vi "SOC_FM Settings Dialog.vi"(8 "error in (no error)":errorcluster, 11 "User Specified":T1={"Hardware Configuration"={"HW Refnum <Replace Me>"="", "Signal Type <Replace Me>"=enum."Sine Wave"}, "Analysis Configuration"={"Statistics"=TRUE}, "New Data Behavior"=enum."Replace", "Calc PPL Path"=path "", "Calc Plugin Class Qualified Name"="", "Calc Configuration String"=""}) -> (0 "error out":errorcluster, 2 "UI Refresh Needed?":bool, 3 "User Specified 2":T1={"Hardware Configuration"={"HW Refnum <Replace Me>"="", "Signal Type <Replace Me>"=enum."Sine Wave"}, "Analysis Configuration"={"Statistics"=TRUE}, "New Data Behavior"=enum."Replace", "Calc PPL Path"=path "", "Calc Plugin Class Qualified Name"="", "Calc Configuration String"=""})   [LabVIEW 2015]
doc: "Dialog for selecting user specified settings."
uses:
  controls/SOC_FM User Specified Data.ctl
  controls/SOC_FM HW Configuration.ctl
  controls/SOC_FM Simulated Signal Type.ctl
  controls/SOC_FM Analysis Configuration.ctl
  controls/SOC_FM New Data Behavior.ctl
panel:
  in  "Calc Configuration String":string
  in  "Calc Plugin Class Qualified Name":string
  in  "Calc PPL Path":path
  in  "Signal Type":u16(ring) items=["Sine Wave", "Square Wave"]
  in  "New Data Behavior":u16(ring) items=["Replace", "Overlay", "Append"]
  in  "Cancel Button":bool
  in  "OK Button":bool
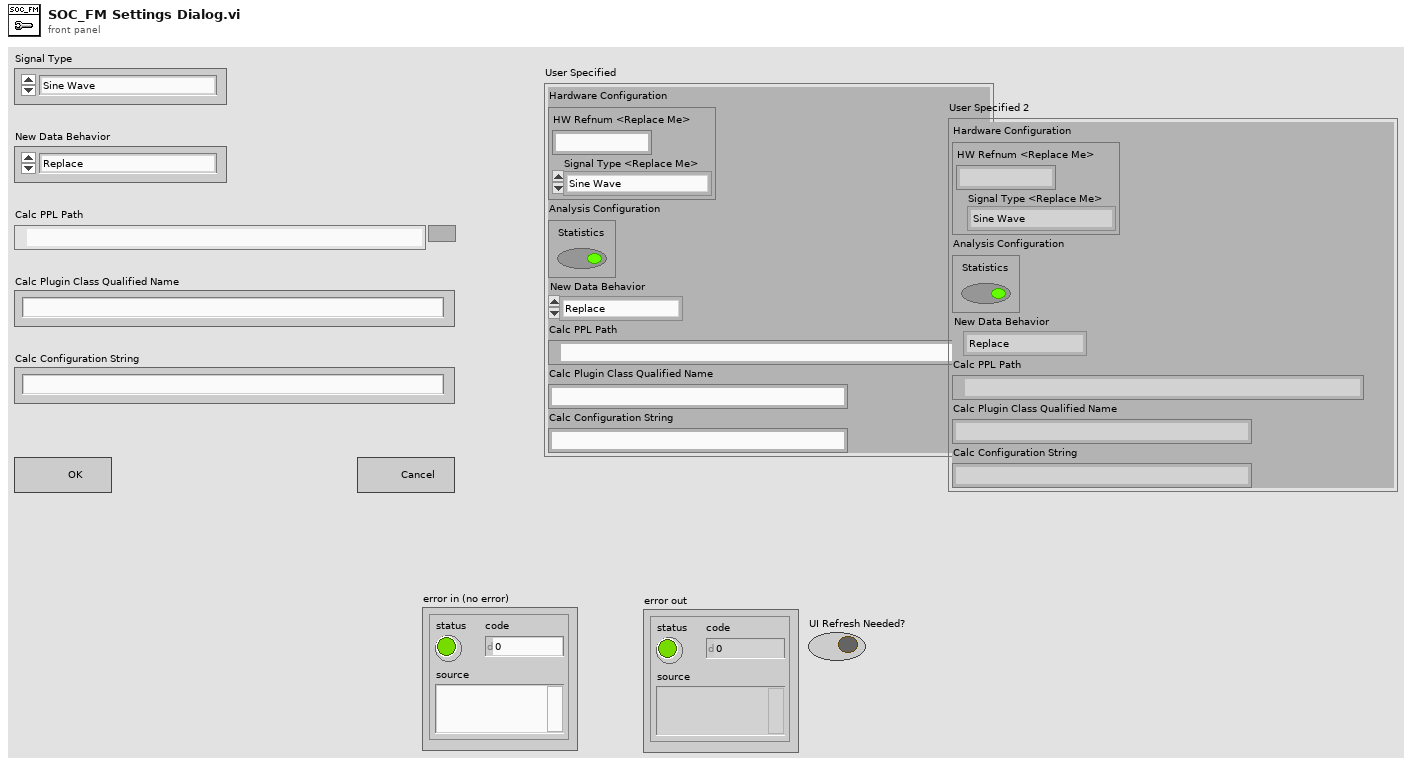
[diagram p1: front panel]
types:
  T1 = typedef "SOC_FM User Specified Data.ctl" = cluster{"Hardware Configuration":T2, "Analysis Configuration":T4, "New Data Behavior":T5, "Calc PPL Path":path, "Calc Plugin Class Qualified Name":string, "Calc Configuration String":string}
  T2 = typedef "SOC_FM HW Configuration.ctl" = cluster{"HW Refnum <Replace Me>":string, "Signal Type <Replace Me>":T3}
  T3 = typedef "SOC_FM Simulated Signal Type.ctl" = enum16{"Sine Wave", "Square Wave"}
  T4 = typedef "SOC_FM Analysis Configuration.ctl" = cluster{"Statistics":bool}
  T5 = typedef "SOC_FM New Data Behavior.ctl" = enum16{"Replace", "Overlay", "Append"}
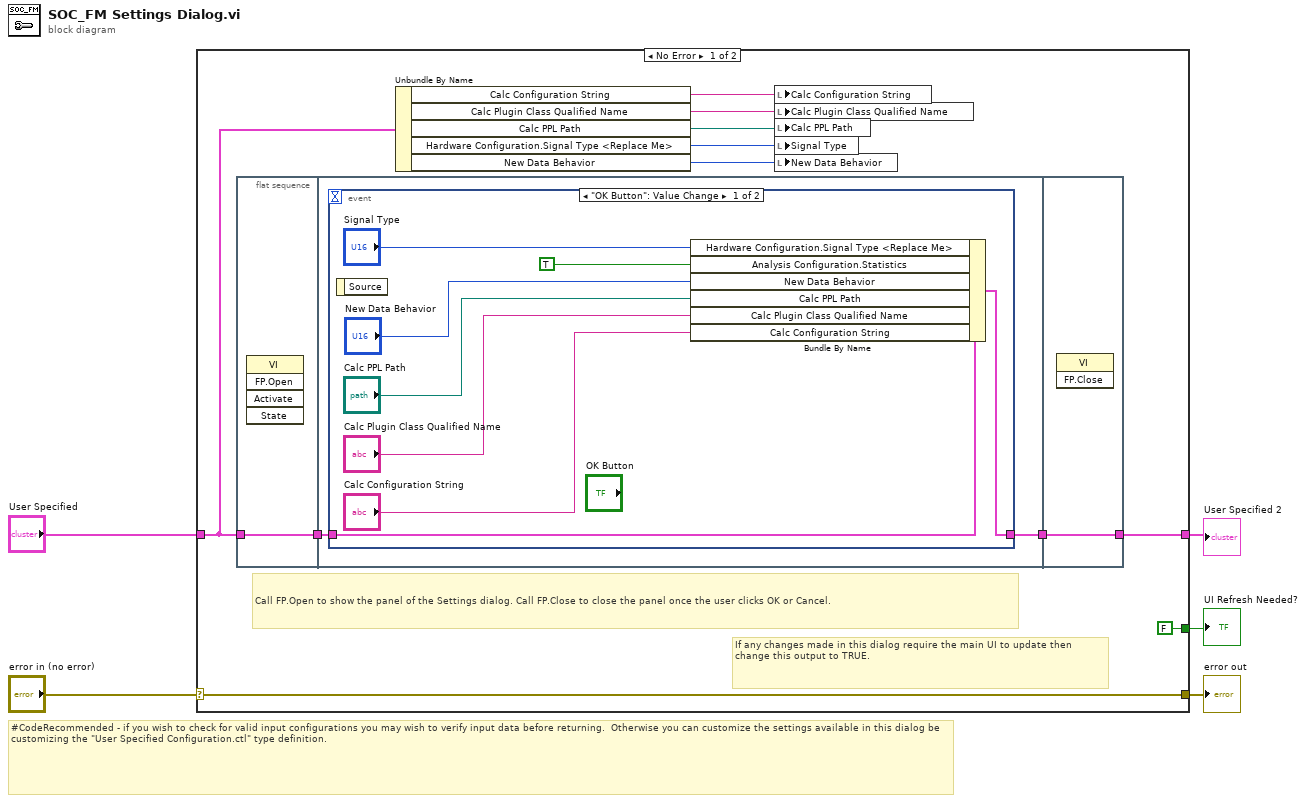
[diagram p0: block diagram]
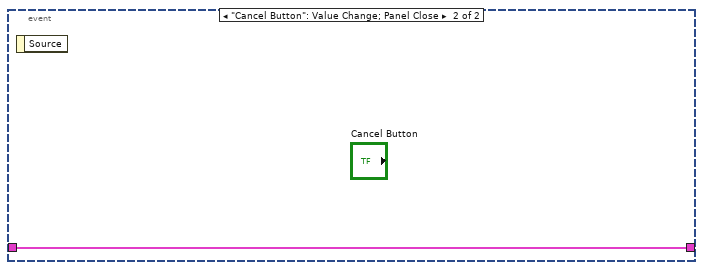
[diagram p2: hidden frame]
diagram:
  # "#CodeRecommended - if you wish to check for valid input configurations you may wish to verify input data before returning.  Otherwise you can customize the settings available in this dialog be customizing the \"User Specified Configuration.ctl\" type definition."
  n1 = case shown="No Error" "error in (no error)" {
    selector: "error in (no error)" -> [w16 w31]
    tunnel: [w16 w31] -> w4
    tunnel: "User Specified" -> [w13 w30]
    tunnel: [w15 w30] -> w1
    tunnel: [FALSE ("UI Refresh Needed?") _] -> w3
    frame No Error {
      # "Call FP.Open to show the panel of the Settings dialog. Call FP.Close to close the panel once the user clicks OK or Cancel."
      # "If any changes made in this dialog require the main UI to update then change this output to TRUE."
      n2 = flat-sequence {
        tunnel: w13 -> [w17]
        tunnel: [w17] -> w10
        tunnel: w10 -> [w18]
        tunnel: [w19] -> w9
        tunnel: [w29] -> w15
        tunnel: w9 -> [w29]
        frame #0 {
          n3 = invoke class="VI" method="FP.Open"() -> ()  [unwired: 5 in, 5 out]
        }
        frame #1 {
          n4 = event shown="[0] \"OK Button\": Value Change" {
            selector: _ -> [_ _]
            dyn-events: _ -> [_ _]
            timeout: _ -> [_ _]
            tunnel: [w26 w28] -> w19
            tunnel: w18 -> [w27 w28]
            event "OK Button": Value Change {
              n5 = event-data() -> ()  [unwired: 1 in, 1 out]
              n6 = Bundle By Name(cluster=w27, "Hardware Configuration.Signal Type <Replace Me>"="Signal Type", "Analysis Configuration.Statistics"=TRUE, "New Data Behavior"="New Data Behavior", "Calc PPL Path"="Calc PPL Path", "Calc Plugin Class Qualified Name"="Calc Plugin Class Qualified Name", "Calc Configuration String"="Calc Configuration String") -> (w26:T1)
            }
            event "Cancel Button": Value Change; Panel Close {
              n7 = event-data() -> ()  [unwired: 1 in, 1 out]
            }
          }
        }
        frame #2 {
          n8 = invoke class="VI" method="FP.Close"() -> ()  [unwired: 3 in, 3 out]
        }
      }
      n9 = Unbundle By Name(w13) -> ("Calc Configuration String"=w7:string, "Calc Plugin Class Qualified Name"=w6:string, "Calc PPL Path"=w8:path, "Hardware Configuration.Signal Type <Replace Me>"=w12:T3, "New Data Behavior"=w11:T5)
      n10 = local write "Calc Configuration String"(w7) -> ()
      n11 = local write "Calc Plugin Class Qualified Name"(w6) -> ()
      n12 = local write "Calc PPL Path"(w8) -> ()
      n13 = local write "Signal Type"(w12) -> ()
      n14 = local write "New Data Behavior"(w11) -> ()
    }
    frame Error {
    }
  }
  "UI Refresh Needed?" <- w3
  "error out" <- w4
  "User Specified 2" <- w1
